vi "Save All Changes in This Project.vi"(8 "error in (no error)":errorcluster, 10 "Exclude Dependencies? (F)":bool, 11 "Project in":refnum<vi>) -> (0 "error out":errorcluster, 3 "Project out":refnum<vi>)   [LabVIEW 2020, in "ADAS_IO_Template_MDO.lvclass"]
doc: "Given a project reference, this VI saves all the VIs and libraries in the project and the project itself. This is equivalent to choosing the File >> Save All (This Project) menu item."
uses:
  ADAS_IO_Template_MDO.lvclass
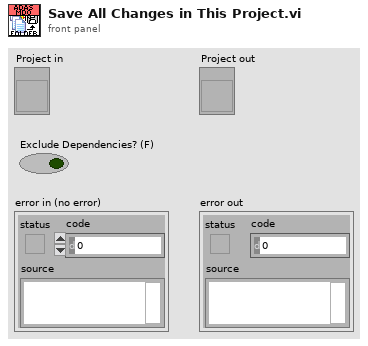
[diagram p1: front panel]
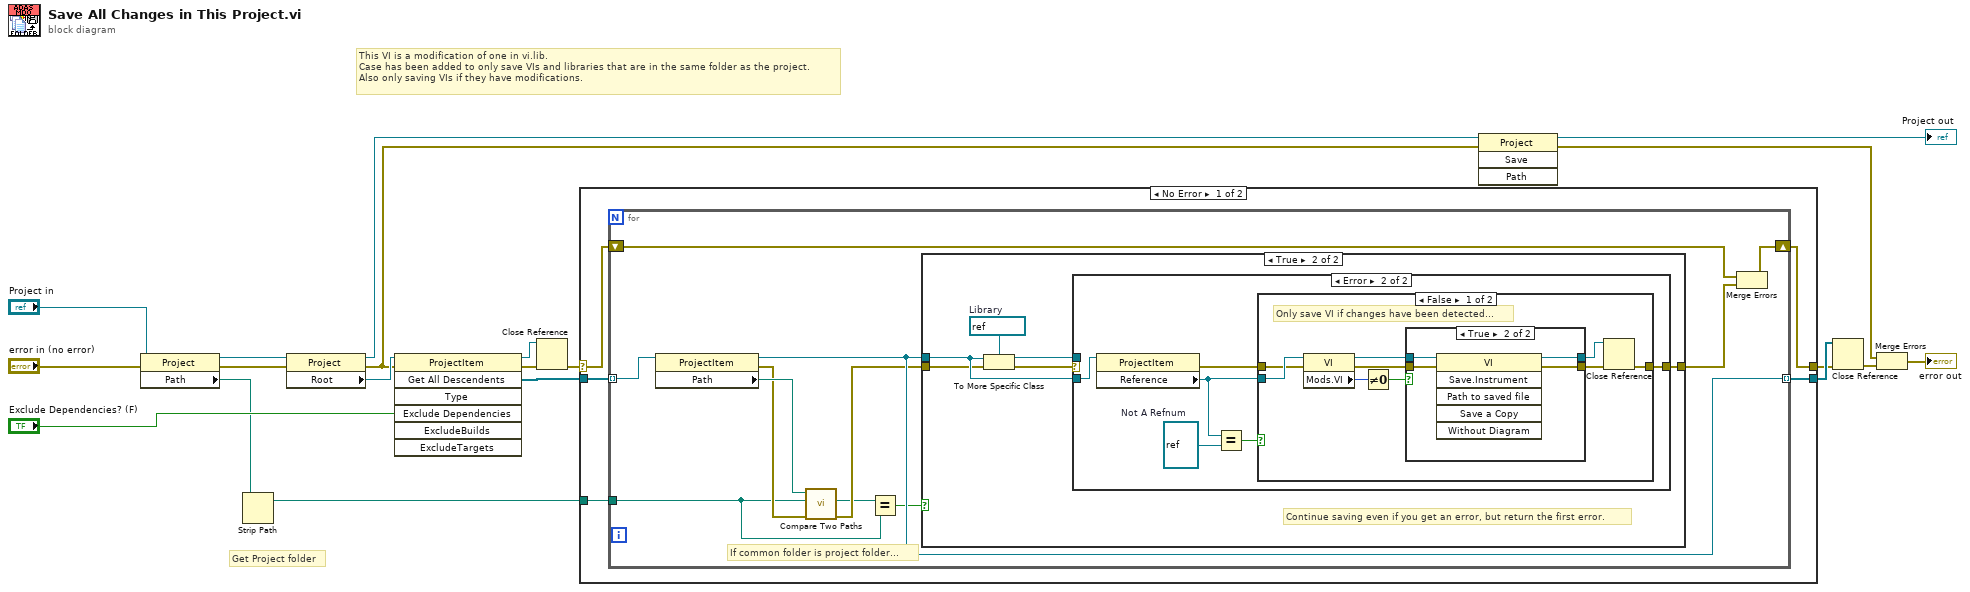
[diagram p0: block diagram]
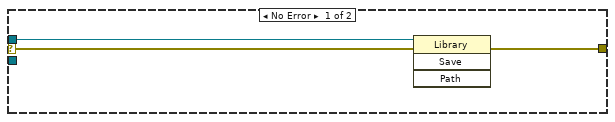
[diagram p3: hidden frame]
diagram:
  # "Get Project folder"
  # "This VI is a modification of one in vi.lib.\nCase has been added to only save VIs and libraries that are in the same folder as the project.\nAlso only saving VIs if they have modifications."
  n1 = property class="Project"(reference="Project in", error in="error in (no error)") -> (reference out=w5:refnum<vi>, error out=w3:errorcluster, "Path"=w2:path)
  n2 = Strip Path(path=w2) -> (stripped path=w1:path)  [unwired: 1 out]
  n3 = property class="Project"(reference=w5, error in=w3) -> (reference out=w16:refnum<vi>, error out=w8:errorcluster, "Root"=w15:refnum<vi>)
  n4 = invoke class="ProjectItem" method="Get All Descendents"(reference=w15, error in=w8, "Exclude Dependencies"="Exclude Dependencies? (F)") -> (reference out=w17:refnum<vi>, error out=w18:errorcluster, "All Descendents"=w19:refnum<vi>[])  [unwired: 4 in, 4 out]
  n5 = Close Reference(reference=w17, error in (no error)=w18) -> (error out=w13:errorcluster)
  n6 = case shown="No Error" w13 {
    selector: w13 -> [w23 w69]
    tunnel: [w25 w68] -> w20
    tunnel: w19 -> [w24 w68]
    tunnel: [w22 w69] -> w12
    tunnel: w1 -> [w21 _]
    frame No Error {
      n7 = for {
        tunnel: w24 -> [w34] mode=indexing
        tunnel: [w33] -> w25 mode=indexing
        shift-right: [w36] -> w22
        shift-left: w23 -> [w32]
        tunnel: w21 -> [w27]
        # "If common folder is project folder..."
        n8 = property class="ProjectItem"(reference=w34) -> (reference out=w33:refnum<vi>, error out=w30:errorcluster, "Path"=w31:path)  [unwired: 1 in]
        n9 = call <vilib>:"Compare Two Paths.vi"("error in (no error)"=w30, "Path 2"=w27, "Path 1"=w31) -> ("error out"=w29:errorcluster, "Common Path"=w28:path)  [unwired: 5 in, 2 out]
        n10 = Equal?(x=w28, y=w27) -> (x = y?=w26:bool)
        n11 = case shown="True" w26 {
          tunnel: [w37 w40] -> w35
          tunnel: w33 -> [_ w39]
          tunnel: w29 -> [w37 w38]
          frame False {
            # "If file path isn't in the project folder, then don't save...."
          }
          frame True {
            w43 = refnum<vi> refnum  # Library
            # "Continue saving even if you get an error, but return the first error."
            n12 = To More Specific Class(target class=w43, reference=w39, error in=w38) -> (specific class reference=w42:refnum<vi>, error out=w41:errorcluster)
            n13 = case shown="Error" w41 {
              selector: w41 -> [w45 _]
              tunnel: w42 -> [w44 _]
              tunnel: [w46 w47] -> w40
              tunnel: w39 -> [_ w51]
              frame No Error {
                n14 = invoke class="Library" method="Save"(reference=w44, error in=w45) -> (error out=w46:errorcluster)  [unwired: 2 in, 3 out]
              }
              frame Error {
                w50 = refnum<vi> refnum  # Not A Refnum
                n15 = property class="ProjectItem"(reference=w51) -> (error out=w52:errorcluster, "Reference"=w48:refnum<vi>)  [unwired: 1 in, 1 out]
                n16 = Equal?(x=w48, y=w50) -> (x = y?=w49:bool)
                n17 = case shown="False" w49 {
                  tunnel: w52 -> [w60 _]
                  tunnel: [w54 _] -> w47
                  tunnel: w48 -> [w61 _]
                  frame False {
                    # "Only save VI if changes have been detected..."
                    n18 = property class="VI"(reference=w61, error in=w60) -> (reference out=w56:refnum<vi>, error out=w58:errorcluster, "Mods.VI"=w59:u64)
                    n19 = Not Equal To 0?(x=w59) -> (x != 0?=w57:bool)
                    n20 = case shown="True" w57 {
                      tunnel: w58 -> [w63 w67]
                      tunnel: w56 -> [w62 w66]
                      tunnel: [w63 w65] -> w55
                      tunnel: [w62 w64] -> w53
                      frame False {
                      }
                      frame True {
                        n21 = invoke class="VI" method="Save.Instrument"(reference=w66, error in=w67) -> (reference out=w64:refnum<vi>, error out=w65:errorcluster)  [unwired: 4 in, 4 out]
                      }
                    }
                    n22 = Close Reference(reference=w53, error in (no error)=w55) -> (error out=w54:errorcluster)
                  }
                  frame True {
                    # "Does not return an error\nif no VI reference available."
                  }
                }
              }
            }
          }
        }
        n23 = Merge Errors(w32, w35) -> (w36:errorcluster)
      }
    }
    frame Error {
    }
  }
  n24 = invoke class="Project" method="Save"(reference=w16, error in=w8) -> (reference out=→"Project out":refnum<vi>, error out=w10:errorcluster)  [unwired: 2 in, 2 out]
  n25 = Close Reference(reference=w20, error in (no error)=w12) -> (error out=w11:errorcluster)
  n26 = Merge Errors(w10, w11) -> (→"error out":errorcluster)
